vi "GetOwner.vi"(6 "error in":errorcluster, 9 "GObject in":refnum<class "GObject.lvclass">) -> (0 "error out":errorcluster, 3 "GObject out":refnum<class "GObject.lvclass">, 4 "Owner":i32)   [LabVIEW 2014, in "GObject.lvclass"]
uses:
  GObject.lvclass
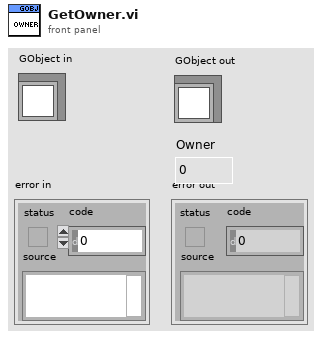
[diagram p1: front panel]
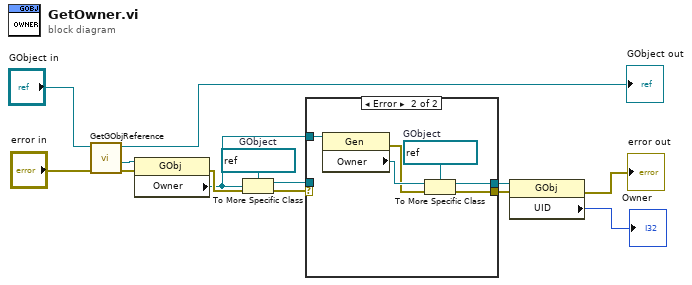
[diagram p0: block diagram]
diagram:
  w5 = refnum<vi> refnum  # GObject
  n1 = call "GetGObjReference.vi"("error in"="error in", "GObject in"="GObject in") -> ("error out"=w11:errorcluster, "reference out"=w12:refnum<vi>, "GObject out"=→"GObject out":refnum<class "GObject.lvclass">)  [unwired: 5 in]
  n2 = property class="GObj"(reference=w12, error in=w11) -> (error out=w4:errorcluster, "Owner"=w1:refnum<vi>)  [unwired: 1 out]
  n3 = To More Specific Class(target class=w5, reference=w1, error in=w4) -> (specific class reference=w2:refnum<vi>, error out=w3:errorcluster)
  n4 = case shown="Error" w3 {
    selector: w3 -> [w15 _]
    tunnel: [w16 w22] -> w8
    tunnel: [w15 w21] -> w7
    tunnel: w2 -> [w16 _]
    tunnel: w1 -> [_ w19]
    frame No Error {
    }
    frame Error {
      w20 = refnum<vi> refnum  # GObject
      n5 = property class="Gen"(reference=w19) -> (error out=w17:errorcluster, "Owner"=w18:refnum<vi>)  [unwired: 1 in, 1 out]
      n6 = To More Specific Class(target class=w20, reference=w18, error in=w17) -> (specific class reference=w22:refnum<vi>, error out=w21:errorcluster)
    }
  }
  n7 = property class="GObj"(reference=w8, error in=w7) -> (error out=→"error out":errorcluster, "UID"=→"Owner":i32)  [unwired: 1 out]
